vi "K_S30_VISA F32.vi"(4 "error in":errorcluster, 6 "Config. Nr.":u8=1, 7 "Address":u8=250) -> (0 "error out":errorcluster, 3 "Configuration":u8 format="%.0b")   [LabVIEW 2012]
panel:
  # "Function 32: Read cofiguration\nV1.0, b.v."
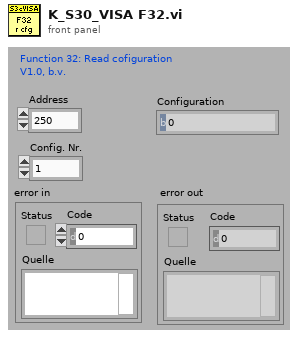
[diagram p1: front panel]
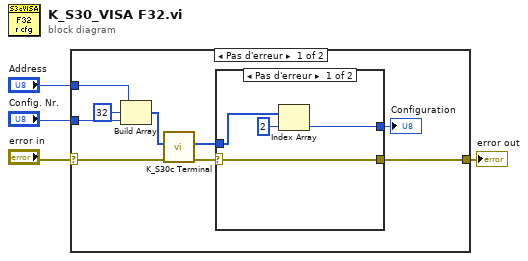
[diagram p0: block diagram]
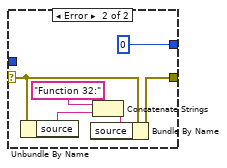
[diagram p2: hidden frame]
diagram:
  n1 = case shown="Pas d'erreur" "error in" {
    selector: "error in" -> [w10 w24]
    tunnel: "Address" -> [w13 _]
    tunnel: [w8 w24] -> w2
    tunnel: "Config. Nr." -> [w6 _]
    frame No Error {
      n2 = Build Array(w13, u8 32 ("Element"), w6) -> (w11:u8[])
      n3 = call "K_S30c Terminal.vi"("error in"=w10, "request"=w11) -> ("error out"=w9:errorcluster, "response"=w7:u8[])  [unwired: 4 in]
      n4 = case shown="Pas d'erreur" w9 {
        selector: w9 -> [w17 w23]
        tunnel: [w17 w21] -> w8
        tunnel: w7 -> [w16 _]
        tunnel: [w14 u8 0] -> w5
        frame No Error {
          n5 = Index Array(array=w16, index=2 ("Index")) -> (element=w14:u8)
        }
        frame Error {
          n6 = Unbundle By Name(w23) -> ("source"=w19:string)
          n7 = Concatenate Strings("Function 32:" ("String"), w19) -> (w22:string)
          n8 = Bundle By Name(cluster=w23, "source"=w22) -> (w21:errorcluster)
        }
      }
      "Configuration" <- w5
    }
    frame Error {
    }
  }
  "error out" <- w2
